vi "Create from CSV Row.vi"(8 "error in (no error)":errorcluster, 11 "CSV Row":string) -> (0 "error out":errorcluster, 3 "Banking Record":refnum<class "Banking Record.lvclass">)   [LabVIEW 2018, in "Banking Record.lvclass"]
uses:
  Banking Record.lvclass
  C:/Users/jtipps/Documents/Filthy-Lucre-Budgetizer/source/support/classes/Transaction/Transaction.lvclass
  <vilib>/Utility/miscctls.llb/LVDateTimeRec.ctl
  Banking Record.lvclass/Banking Record.ctl
  Transaction/Transaction.lvclass
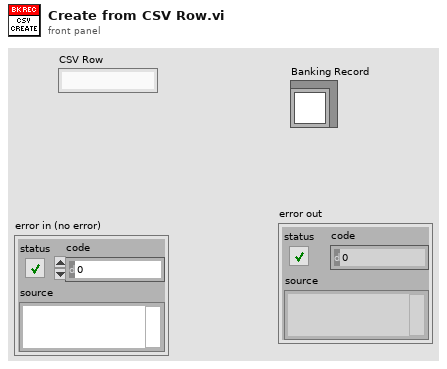
[diagram p1: front panel]
types:
  T1 = typedef "LVDateTimeRec.ctl" = cluster{"fractional second":dbl, "second":i32, "minute":i32, "hour":i32, "day of month":i32, "month":i32, "year":i32, "day of week":i32, "day of year":i32, "DST":i32}
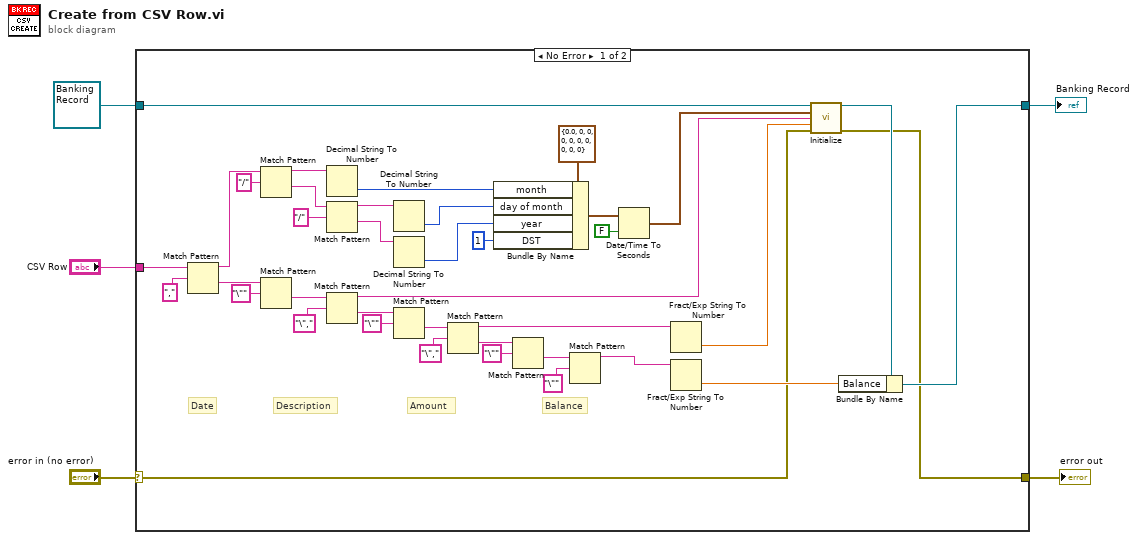
[diagram p0: block diagram]
diagram:
  n1 = case shown="No Error" "error in (no error)" {
    selector: "error in (no error)" -> [w7 w46]
    tunnel: [w44 w45] -> w5
    tunnel: "CSV Row" -> [w16 _]
    tunnel: [w6 w46] -> w2
    tunnel: refnum<class "Banking Record.lvclass"> refnum ("Banking Record.lvclass") -> [w12 w45]
    frame No Error {
      # "Balance"
      # "Amount"
      # "Description"
      # "Date"
      n2 = Match Pattern(string=w16, regular expression=",") -> (before substring=w15:string, after substring=w43:string)  [unwired: 3 out]
      n3 = Match Pattern(string=w15, regular expression="/") -> (before substring=w26:string, after substring=w24:string)  [unwired: 3 out]
      n4 = Match Pattern(string=w43, regular expression="\"") -> (after substring=w41:string)  [unwired: 4 out]
      n5 = Decimal String To Number(string=w26) -> (number=w23:i32)  [unwired: 2 in, 1 out]
      n6 = Match Pattern(string=w24, regular expression="/") -> (before substring=w22:string, after substring=w20:string)  [unwired: 3 out]
      n7 = Match Pattern(string=w41, regular expression="\",") -> (before substring=w9:string, after substring=w36:string)  [unwired: 3 out]
      n8 = Decimal String To Number(string=w22) -> (number=w21:i32)  [unwired: 2 in, 1 out]
      n9 = Decimal String To Number(string=w20) -> (number=w19:i32)  [unwired: 2 in, 1 out]
      n10 = Match Pattern(string=w36, regular expression="\"") -> (after substring=w38:string)  [unwired: 4 out]
      n11 = Match Pattern(string=w38, regular expression="\",") -> (before substring=w31:string, after substring=w32:string)  [unwired: 3 out]
      n12 = Bundle By Name(cluster=T1 {"fractional second"=0.0, "second"=0, "minute"=0, "hour"=0, "day of month"=0, "month"=0, "year"=0, "day of week"=0, "day of year"=0, "DST"=0} ("date time rec"), "month"=w23, "day of month"=w21, "year"=w19, "DST"=1) -> (w29:T1)
      n13 = Match Pattern(string=w32, regular expression="\"") -> (after substring=w34:string)  [unwired: 4 out]
      n14 = Match Pattern(string=w34, regular expression="\"") -> (before substring=w30:string)  [unwired: 4 out]
      n15 = Date/Time To Seconds(1:FALSE ("is UTC (F)"), 2:w29) -> (0:w10:timestamp)
      n16 = Fract/Exp String To Number(string=w31) -> (number=w8:dbl)  [unwired: 3 in, 1 out]
      n17 = Fract/Exp String To Number(string=w30) -> (number=w18:dbl)  [unwired: 3 in, 1 out]
      n18 = call "Initialize.vi"("Transaction in"=w12, "Date"=w10, "Description"=w9, "Amount"=w8, "error in (no error)"=w7) -> ("Transaction out"=w11:refnum<class "Banking Record.lvclass">, "error out"=w6:errorcluster)  [unwired: 9 in]
      n19 = Bundle By Name(cluster=w11, "Balance"=w18) -> (w44:refnum<class "Banking Record.lvclass">)
    }
    frame Error {
    }
  }
  "Banking Record" <- w5
  "error out" <- w2
